vi "getParameters.vi"(8 "error in (no error)":errorcluster, 11 "IDataRule in":refnum<class "IDataRule.lvclass">) -> (0 "error out":errorcluster, 2 "Parameters out":refnum<class "IDict.lvclass">, 3 "IDataRule out":refnum<class "IDataRule.lvclass">)   [LabVIEW 2022 SP3, in "openDAQ.lvlib" / "IBaseObject.lvlib" / "IDataRule.lvlib" / "IDataRule.lvclass"]
uses:
  <instrlib>/openDAQ/Public/Classes/IDataRule/IDataRule.lvclass
  <instrlib>/openDAQ/Public/Classes/IDataRule/IDataRule.lvclass/IDataRule.ctl
  <instrlib>/openDAQ/Public/Classes/daqCoreTypes/IDict/IDict.lvclass
  <instrlib>/openDAQ/Binaries/Windows/x86/copendaq32.dll
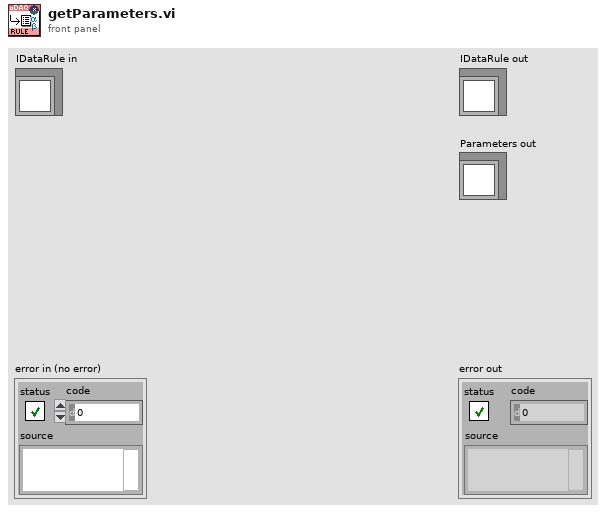
[diagram p1: front panel]
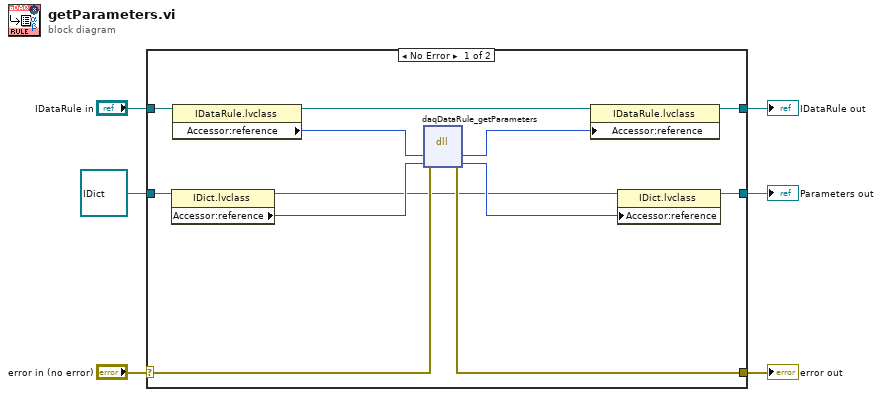
[diagram p0: block diagram]
diagram:
  n1 = case shown="No Error" "error in (no error)" {
    selector: "error in (no error)" -> [w16 w21]
    tunnel: [w15 w21] -> w5
    tunnel: [w11 w20] -> w3
    tunnel: "IDataRule in" -> [w17 w20]
    tunnel: refnum<class "IDict.lvclass"> refnum ("openDAQ.lvlib:daqCoreTypes.lvlib:IDict.lvclass") -> [w10 w19]
    tunnel: [w7 w19] -> w1
    frame No Error {
      n2 = property class="IDict.lvclass"(reference=w10) -> (reference out=w8:refnum<class "IDict.lvclass">, "Accessor:reference"=w9:i64)  [unwired: 1 in, 1 out]
      n3 = property class="IDataRule.lvclass"(reference=w17) -> (reference out=w12:refnum<class "IDataRule.lvclass">, "Accessor:reference"=w14:i64)  [unwired: 1 in, 1 out]
      n4 = dll-call lib="C:/Program Files (x86)/National Instruments/LabVIEW 2022/instr.lib/openDAQ/Binaries/Windows/x86/copendaq*.*" fn="daqDataRule_getParameters"(error in=w16, "dataRule"=w14, "parameters"=w9) -> (error out=w15:errorcluster, "dataRule"=w13:i64, "parameters"=w18:i64)  [unwired: 3 in, 1 out]
      n5 = property class="IDataRule.lvclass"(reference=w12, "Accessor:reference"=w13) -> (reference out=w11:refnum<class "IDataRule.lvclass">)  [unwired: 1 in, 1 out]
      n6 = property class="IDict.lvclass"(reference=w8, "Accessor:reference"=w18) -> (reference out=w7:refnum<class "IDict.lvclass">)  [unwired: 1 in, 1 out]
    }
    frame Error {
    }
  }
  "error out" <- w5
  "IDataRule out" <- w3
  "Parameters out" <- w1
